vi "柱塞泵操作的步数 (子VI).vi"(8 "Error in":errorcluster caption="Error in (no error)", 10 "柱塞泵步数":u16, 11 "仪器":enum16{"", "氨氮", "总磷", "总氮", "CODMn", "CODCr"}(ring)=enum."氨氮") -> (0 "error out":errorcluster)   [LabVIEW 2016, in "质控单元.lvlib"]
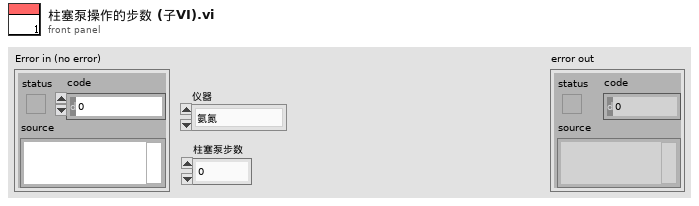
[diagram p1: front panel]
types:
  T1 = cluster{"仪器":enum16{"", "氨氮", "总磷", "总氮", "CODMn", "CODCr"}, "starting address":u16, "value":u16}
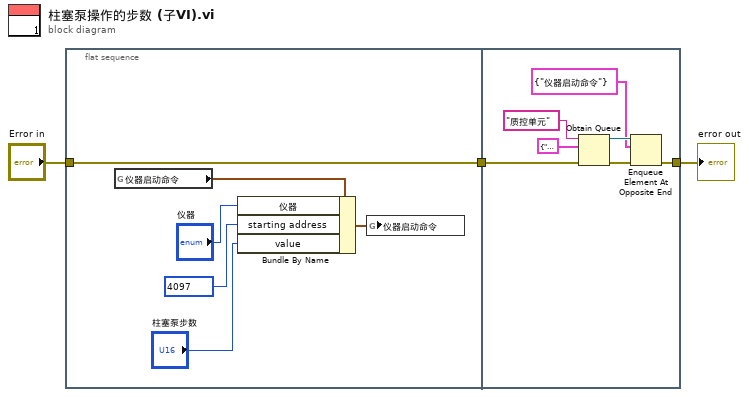
[diagram p0: block diagram]
diagram:
  n1 = flat-sequence {
    tunnel: "Error in" -> [w7]
    tunnel: [w7] -> w3
    tunnel: w3 -> [w11]
    tunnel: [w10] -> w2
    frame #0 {
      n2 = global read "质控内部交互全局.vi" "仪器启动命令"() -> (w8:T1)
      n3 = Bundle By Name(cluster=w8, "仪器"="仪器", "starting address"=u16 4097, "value"="柱塞泵步数") -> (w9:T1)
      n4 = global write "质控内部交互全局.vi" "仪器启动命令"(w9) -> ()
    }
    frame #1 {
      n5 = Obtain Queue(name (unnamed)="质控单元" ("名称（未命名）"), element data type=cluster{"命令":string} {"命令"="启用模块"} ("元素"), error in (no error)=w11) -> (queue out=w14:refnum<queue>, error out=w13:errorcluster)  [unwired: 2 in, 1 out]
      n6 = Enqueue Element At Opposite End(queue=w14, element=cluster{"命令":string} {"命令"="仪器启动命令"} ("元素"), error in (no error)=w13) -> (error out=w10:errorcluster)  [unwired: 1 in, 2 out]
    }
  }
  "error out" <- w2
